vi "Sample_EL6910Diagnostics.vi"() -> ()   [LabVIEW 2022 SP3, in "Safety_Library.lvlib"]
uses:
  Safety_Library.lvlib
  TypeDefs/FSoEConnectionInfoData.ctl
  TypeDefs/DeviceInfoData.ctl
  TypeDefs/FSLogicInputs.ctl
  TypeDefs/TwinSAFEGroupInfoData.ctl
  ADS/ADS_Library.lvlib
panel:
  in  "stop":bool
  out "output cluster 5":T2
  out "output cluster 4":cluster{"SymbolName":string, "FSLogic":T3}
  out "output cluster 3":cluster{"SymbolName":string, "Cluster":T4} {"Cluster"."Project CRC" format="%x"}
  out "output cluster 2":cluster{"SymbolName":string, "InfoData":T5}
  out "output cluster":cluster{"SymbolName":string, "InfoData":T5}
  out "error out":errorcluster
  out "Read status?":bool[](array[boolean])
  in  "String":string="<PortInfo><Inputs><SymbolControlItems /></Inputs><Outputs><SymbolControlItems><SymbolControlItem GroupName=\"ADS Read\" GroupDescription=\"Parameters for ADS Read command\"><Parameters><Parameter Name=\"Name\">Term 5 (EL6910).Connection Info Data.Message_2 Info Data</Parameter><Parameter Name=\"SymbolName\">Term 5 (EL6910).Connection Info Data.Message_2 Info Data</Parameter><Parameter Name=\"SymbolType\">INFODATA_2542655572</Parameter><Parameter Name=\"SymbolGuid\"></Parameter><Parameter Name=\"AmsNetId\">192.168.80.50.1.1</Parameter><Parameter Name=\"Port\">27908</Parameter><Parameter Name=\"IndexGroup\">#x0</Parameter><Parameter Name=\"IndexOffset\">#x0</Parameter><Parameter Name=\"BitSize\">24</Parameter><Parameter Name=\"CycleTime [ms]\">10</Parameter><Parameter Name=\"Transmode\">3</Parameter><Parameter Name=\"Timeout [ms]\">1000</Parameter><Parameter Name=\"TCBufferSize [Samples]\">10</Parameter><Parameter Name=\"LVBufferSize [Samples]\">50</Parameter><Parameter Name=\"Expected min delay [ms]\">500</Parameter></Parameters></SymbolControlItem><SymbolControlItem GroupName=\"ADS Read\" GroupDescription=\"Parameters for ADS Read command\"><Parameters><Parameter Name=\"Name\">Term 5 (EL6910).Connection Info Data.Message_3 Info Data</Parameter><Parameter Name=\"SymbolName\">Term 5 (EL6910).Connection Info Data.Message_3 Info Data</Parameter><Parameter Name=\"SymbolType\">INFODATA_162409835</Parameter><Parameter Name=\"SymbolGuid\"></Parameter><Parameter Name=\"AmsNetId\">192.168.80.50.1.1</Parameter><Parameter Name=\"Port\">27908</Parameter><Parameter Name=\"IndexGroup\">#x0</Parameter><Parameter Name=\"IndexOffset\">#x0</Parameter><Parameter Name=\"BitSize\">24</Parameter><Parameter Name=\"CycleTime [ms]\">10</Parameter><Parameter Name=\"Transmode\">3</Parameter><Parameter Name=\"Timeout [ms]\">1000</Parameter><Parameter Name=\"TCBufferSize [Samples]\">10</Parameter><Parameter Name=\"LVBufferSize [Samples]\">50</Parameter><Parameter Name=\"Expected min delay [ms]\">500</Parameter></Parameters></SymbolControlItem><SymbolControlItem GroupName=\"ADS Read\" GroupDescription=\"Parameters for ADS Read command\"><Parameters><Parameter Name=\"Name\">Term 5 (EL6910).Device Info Data</Parameter><Parameter Name=\"SymbolName\">Term 5 (EL6910).Device Info Data</Parameter><Parameter Name=\"SymbolType\">Device Info Data_1_TYPE</Parameter><Parameter Name=\"SymbolGuid\"></Parameter><Parameter Name=\"AmsNetId\">192.168.80.50.1.1</Parameter><Parameter Name=\"Port\">27908</Parameter><Parameter Name=\"IndexGroup\">#x0</Parameter><Parameter Name=\"IndexOffset\">#x0</Parameter><Parameter Name=\"BitSize\">48</Parameter><Parameter Name=\"CycleTime [ms]\">10</Parameter><Parameter Name=\"Transmode\">3</Parameter><Parameter Name=\"Timeout [ms]\">1000</Parameter><Parameter Name=\"TCBufferSize [Samples]\">10</Parameter><Parameter Name=\"LVBufferSize [Samples]\">50</Parameter><Parameter Name=\"Expected min delay [ms]\">500</Parameter></Parameters></SymbolControlItem><SymbolControlItem GroupName=\"ADS Read\" GroupDescription=\"Parameters for ADS Read command\"><Parameters><Parameter Name=\"Name\">Term 5 (EL6910).FSLOGIC Inputs</Parameter><Parameter Name=\"SymbolName\">Term 5 (EL6910).FSLOGIC Inputs</Parameter><Parameter Name=\"SymbolType\">FSLOGIC Inputs_1_TYPE</Parameter><Parameter Name=\"SymbolGuid\"></Parameter><Parameter Name=\"AmsNetId\">192.168.80.50.1.1</Parameter><Parameter Name=\"Port\">27908</Parameter><Parameter Name=\"IndexGroup\">#x0</Parameter><Parameter Name=\"IndexOffset\">#x0</Parameter><Parameter Name=\"BitSize\">16</Parameter><Parameter Name=\"CycleTime [ms]\">10</Parameter><Parameter Name=\"Transmode\">3</Parameter><Parameter Name=\"Timeout [ms]\">1000</Parameter><Parameter Name=\"TCBufferSize [Samples]\">10</Parameter><Parameter Name=\"LVBufferSize [Samples]\">50</Parameter><Parameter Name=\"Expected min delay [ms]\">500</Parameter></Parameters></SymbolControlItem><SymbolControlItem GroupName=\"ADS Read\" GroupDescription=\"Parameters for ADS Read command\"><Parameters><Parameter Name=\"Name\">Term 5 (EL6910).TwinSAFE Group Info Data.TwinSafeGroup1 Info Data</Parameter><Parameter Name=\"SymbolName\">Term 5 (EL6910).TwinSAFE Group Info Data.TwinSafeGroup1 Info Data</Parameter><Parameter Name=\"SymbolType\">INFODATA_GRP_3</Parameter><Parameter Name=\"SymbolGuid\"></Parameter><Parameter Name=\"AmsNetId\">192.168.80.50.1.1</Parameter><Parameter Name=\"Port\">27908</Parameter><Parameter Name=\"IndexGroup\">#x0</Parameter><Parameter Name=\"IndexOffset\">#x0</Parameter><Parameter Name=\"BitSize\">16</Parameter><Parameter Name=\"CycleTime [ms]\">10</Parameter><Parameter Name=\"Transmode\">3</Parameter><Parameter Name=\"Timeout [ms]\">1000</Parameter><Parameter Name=\"TCBufferSize [Samples]\">10</Parameter><Parameter Name=\"LVBufferSize [Samples]\">50</Parameter><Parameter Name=\"Expected min delay [ms]\">500</Parameter></Parameters></SymbolControlItem></SymbolControlItems></Outputs></PortInfo>"
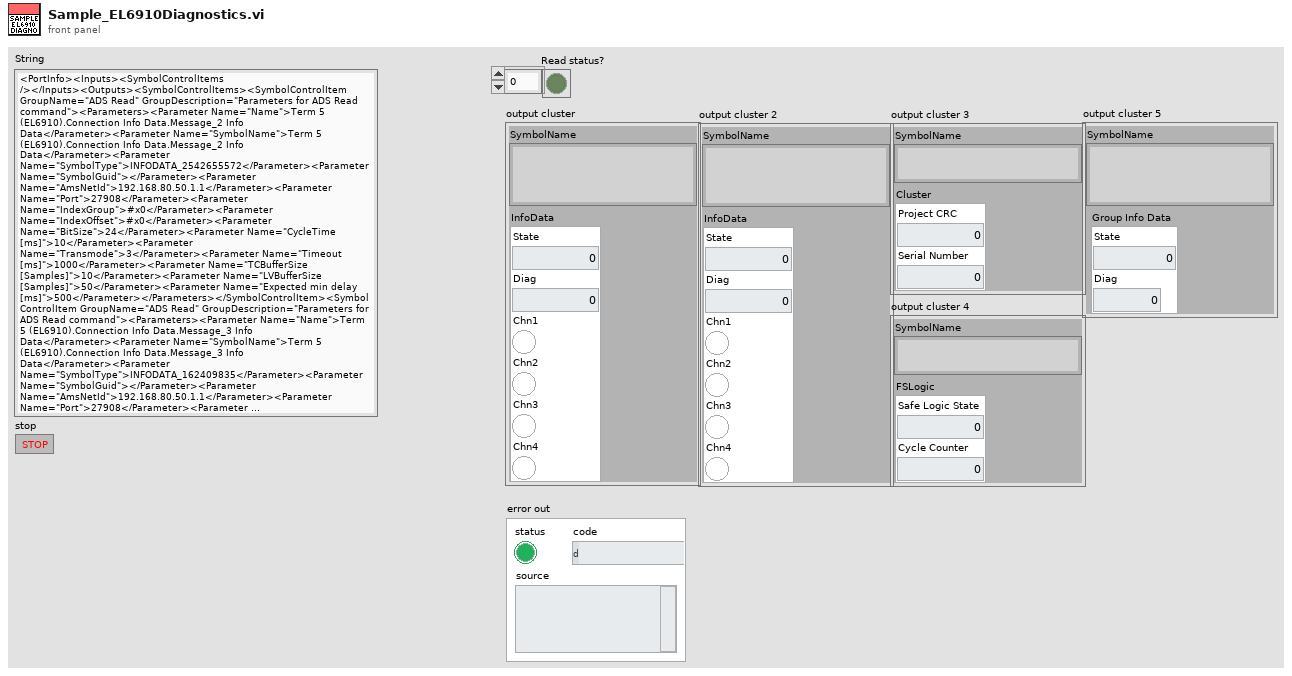
[diagram p1: front panel]
types:
  T1 = typedef "Safety_Library.lvlib/TwinSAFEGroupInfoData.ctl" = cluster{"State":u8, "Diag":u8}
  T2 = cluster{"SymbolName":string, "Group Info Data":T1}
  T3 = typedef "Safety_Library.lvlib/FSLogicInputs.ctl" = cluster{"Safe Logic State":u8, "Cycle Counter":u8}
  T4 = typedef "Safety_Library.lvlib/DeviceInfoData.ctl" = cluster{"Project CRC":u16, "Serial Number":u32}
  T5 = typedef "Safety_Library.lvlib/FSoEConnectionInfoData.ctl" = cluster{"State":dbl, "Diag":dbl, "Chn1":bool, "Chn2":bool, "Chn3":bool, "Chn4":bool}
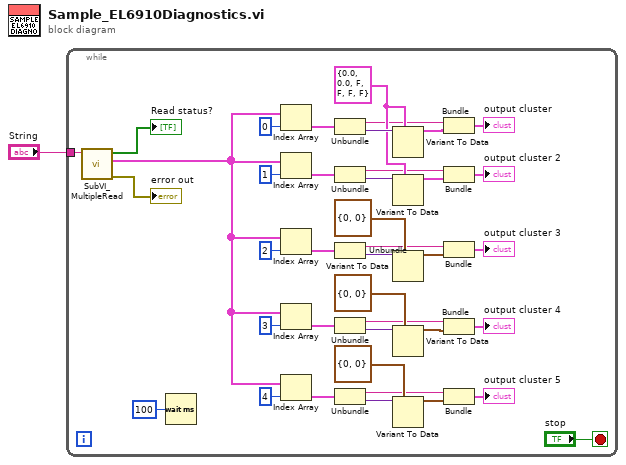
[diagram p0: block diagram]
diagram:
  n1 = while {
    tunnel: "String" -> [w41]
    stop <- "stop" stop-if-true
    w22 = T5 {"State"=0.0, "Diag"=0.0, "Chn1"=FALSE, "Chn2"=FALSE, "Chn3"=FALSE, "Chn4"=FALSE} ("InfoData")
    n2 = call "SubVI_MultipleRead.vi"("String"=w41) -> ("error out"=→"error out":errorcluster, "Data"=w33:cluster{"SymbolName":string, "RData":variant}[], "Read status?"=→"Read status?":bool[])  [unwired: 8 in]
    n3 = Wait (ms)(milliseconds to wait=u32 100) -> ()  [unwired: 1 out]
    n4 = Index Array(array=w33, index=0) -> (element=w32:cluster{"SymbolName":string, "RData":variant})
    n5 = Index Array(array=w33, index=1) -> (element=w31:cluster{"SymbolName":string, "RData":variant})
    n6 = Index Array(array=w33, index=2) -> (element=w30:cluster{"SymbolName":string, "RData":variant})
    n7 = Index Array(array=w33, index=3) -> (element=w29:cluster{"SymbolName":string, "RData":variant})
    n8 = Index Array(array=w33, index=4) -> (element=w28:cluster{"SymbolName":string, "RData":variant})
    n9 = Unbundle(w32) -> ("SymbolName"=w18:string, "RData"=w27:variant)
    n10 = Unbundle(w31) -> ("SymbolName"=w16:string, "RData"=w26:variant)
    n11 = Unbundle(w30) -> ("SymbolName"=w15:string, "RData"=w23:variant)
    n12 = Unbundle(w29) -> ("SymbolName"=w14:string, "RData"=w24:variant)
    n13 = Unbundle(w28) -> ("SymbolName"=w13:string, "RData"=w25:variant)
    n14 = Variant To Data(type=w22, Variant=w27) -> (data=w17:T5)  [unwired: 1 in, 1 out]
    n15 = Variant To Data(type=w22, Variant=w26) -> (data=w12:T5)  [unwired: 1 in, 1 out]
    n16 = Variant To Data(type=T4 {"Project CRC"=0, "Serial Number"=0} ("Cluster"), Variant=w23) -> (data=w11:T4)  [unwired: 1 in, 1 out]
    n17 = Variant To Data(type=T3 {"Safe Logic State"=0, "Cycle Counter"=0} ("FSLogic"), Variant=w24) -> (data=w10:T3)  [unwired: 1 in, 1 out]
    n18 = Variant To Data(type=T1 {"State"=0, "Diag"=0} ("Group Info Data"), Variant=w25) -> (data=w9:T1)  [unwired: 1 in, 1 out]
    n19 = Bundle("SymbolName"=w18, "InfoData"=w17) -> (→"output cluster":cluster{"SymbolName":string, "InfoData":T5})  [unwired: 1 in]
    n20 = Bundle("SymbolName"=w16, "InfoData"=w12) -> (→"output cluster 2":cluster{"SymbolName":string, "InfoData":T5})  [unwired: 1 in]
    n21 = Bundle("SymbolName"=w15, "Cluster"=w11) -> (→"output cluster 3":cluster{"SymbolName":string, "Cluster":T4})  [unwired: 1 in]
    n22 = Bundle("SymbolName"=w14, "FSLogic"=w10) -> (→"output cluster 4":cluster{"SymbolName":string, "FSLogic":T3})  [unwired: 1 in]
    n23 = Bundle("SymbolName"=w13, "Group Info Data"=w9) -> (→"output cluster 5":T2)  [unwired: 1 in]
  }
